vi "Delete Last Element.vi"(0 "Variant (Cluster) in":variant, 11 "error in (no error)":errorcluster) -> (4 "Variant (Cluster) out":variant, 6 "Name":string, 8 "element":variant, 15 "error out":errorcluster)   [LabVIEW 2017, in "Advanced Variant Tools.lvlib"]
uses:
  Advanced Variant Tools.lvlib
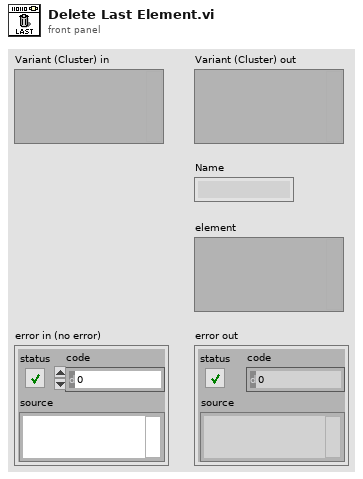
[diagram p1: front panel]
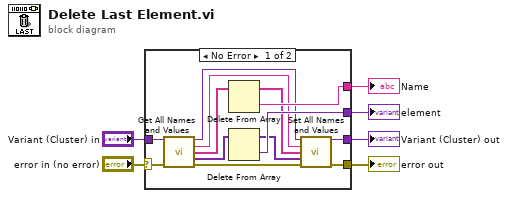
[diagram p0: block diagram]
diagram:
  n1 = case shown="No Error" "error in (no error)" {
    selector: "error in (no error)" -> [w19 w20]
    tunnel: [w16 w20] -> w5
    tunnel: [w15 w21] -> w4
    tunnel: "Variant (Cluster) in" -> [w14 w21]
    tunnel: [w12 _] -> w2
    tunnel: [w11 _] -> w1
    frame No Error {
      n2 = call "Get All Names and Values.vi"("Variant (Cluster) In"=w14, "error in"=w19) -> ("Variant (Cluster) Out"=w7:variant, "Name"=w8:string, "Element Names"=w13:string[], "Values"=w18:variant[], "error out"=w17:errorcluster)  [unwired: 9 in]
      n3 = Delete From Array(array=w13) -> (deleted portion=w12:string, array with subset deleted=w10:string[])  [unwired: 2 in]
      n4 = Delete From Array(array=w18) -> (deleted portion=w11:variant, array with subset deleted=w9:variant[])  [unwired: 2 in]
      n5 = call "Set All Names and Values.vi"("Variant (Cluster) In"=w7, "Name"=w8, "Element Names"=w10, "values"=w9, "error in"=w17) -> ("Variant (Cluster) Out"=w15:variant, "error out"=w16:errorcluster)  [unwired: 9 in]
    }
    frame Error {
    }
  }
  "Variant (Cluster) out" <- w4
  "error out" <- w5
  "element" <- w1
  "Name" <- w2
